vi "Get Torque.vi"(0 "reference in":refnum<class "SmartMotor.lvclass">, 5 "error in (no error)":errorcluster) -> (14 "reference out":refnum<class "SmartMotor.lvclass">, 17 "Motor Torque":i32, 18 "Absolute Motor Torque (Filtered)":dbl, 19 "error out":errorcluster)   [LabVIEW 2017, in "SmartMotor.lvclass"]
uses:
  SmartMotor.lvclass
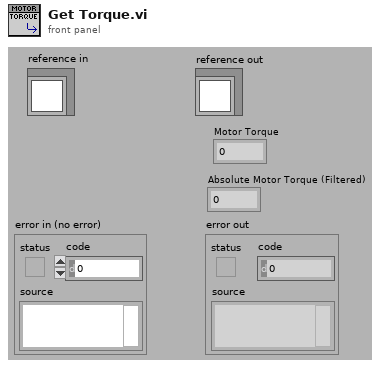
[diagram p1: front panel]
types:
  T1 = typedef "SmartMotor.lvclass/ObjectAttributes.ctl" = cluster{"SmartMotor Chain VISA Resource":refnum<visa-resource-name>, "SmartMotor Chain Address":i16, "Motor Absolute Position":i32, "Motor Relative Position":i32, "Motor Torque":i32, "Motor Voltage":i32, "Screwdriver Engaged":bool, "Screwdriver Torque Limit":i32, "Torque Monitor On/Off Status":bool, "Torque Monitor VI Reference":refnum<vi>, "Absolute Motor Torque (Filtered)":dbl, "SmartMotor Status":T2, "SmartMotor Error":T3}
  T2 = typedef "SmartMotor.lvclass/SmartMotor Status.ctl" = enum8{"Stopped", "Moving"}
  T3 = typedef "SmartMotor.lvclass/SmartMotor Error.ctl" = enum8{"None", "Read Error", "Low Voltage"}
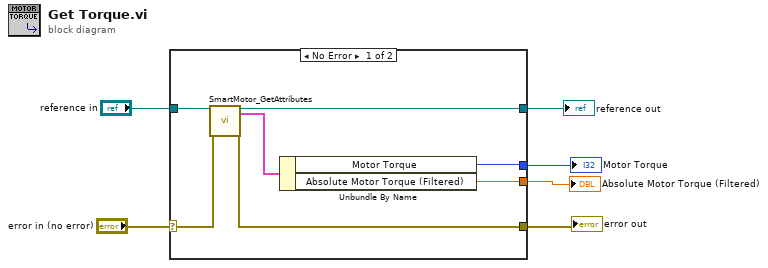
[diagram p0: block diagram]
diagram:
  n1 = case shown="No Error" "error in (no error)" {
    selector: "error in (no error)" -> [w13 w15]
    tunnel: [w11 w15] -> w5
    tunnel: [w9 w14] -> w3
    tunnel: "reference in" -> [w10 w14]
    tunnel: [w8 _] -> w2
    tunnel: [w7 _] -> w1
    frame No Error {
      n2 = call "SmartMotor_GetAttributes.vi"("reference in"=w10, "error in (no error)"=w13) -> ("reference out"=w9:refnum<class "SmartMotor.lvclass">, "Data"=w12:T1, "error out"=w11:errorcluster)  [unwired: 14 in, 1 out]
      n3 = Unbundle By Name(w12) -> ("Motor Torque"=w8:i32, "Absolute Motor Torque (Filtered)"=w7:dbl)
    }
    frame Error {
    }
  }
  "error out" <- w5
  "reference out" <- w3
  "Motor Torque" <- w2
  "Absolute Motor Torque (Filtered)" <- w1
